vi "SwerveChooseBestAngle.vi"(6 "Current Angle":dbl format="%#_13g", 8 "Target Angle":dbl format="%#_13g", 11 "Power In":dbl) -> (0 "Setpoint Angle":dbl format="%_4g", 2 "Power Out":dbl)   [LabVIEW 2020]
doc: "Based on the Current Angle and the Goal Angle, this VI calulates the signed angular distance. Taking into account the option to invert the direction of the swerve drive motor and always picking the shortest travel distance. The hysteresis prevents undesirable vacillation between angle choices."
panel:
  # "(deg) [-180,+180]"
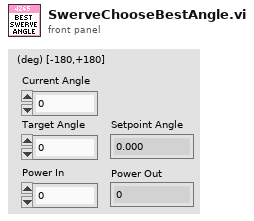
[diagram p1: front panel]
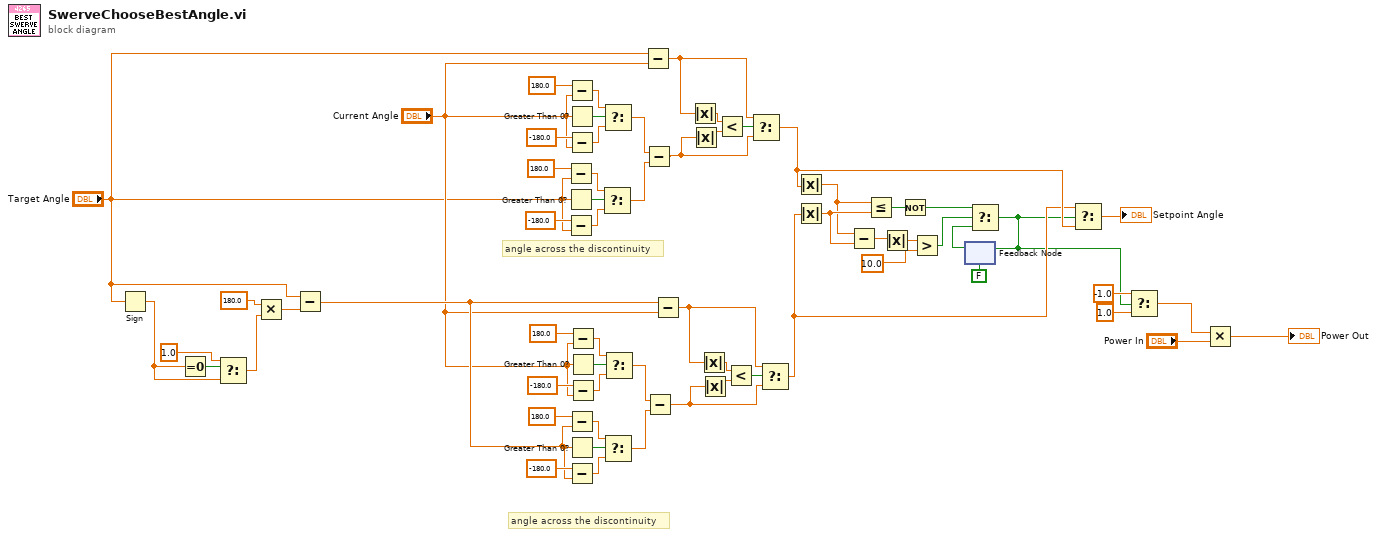
[diagram p0: block diagram]
diagram:
  # "angle across the discontinuity"
  # "angle across the discontinuity"
  n1 = Sign(1:"Target Angle") -> (0:w14:dbl)
  n2 = Equal To 0?(x=w14) -> (x = 0?=w15:bool)
  n3 = Select(t=1.0, s=w15, f=w14) -> (s? t:f=w11:dbl)
  n4 = Multiply(x=180.0 ("y"), y=w11) -> (x*y=w62:dbl)
  n5 = Subtract(x="Target Angle", y=w62) -> (x-y=w36:dbl)
  n6 = Subtract(x=180.0, y="Target Angle") -> (x-y=w24:dbl)
  n7 = Greater Than 0?(x="Target Angle") -> (x > 0?=w26:bool)
  n8 = Subtract(x=-180.0, y="Target Angle") -> (x-y=w22:dbl)
  n9 = Subtract(x=180.0, y="Current Angle") -> (x-y=w29:dbl)
  n10 = Greater Than 0?(x="Current Angle") -> (x > 0?=w31:bool)
  n11 = Subtract(x=-180.0, y="Current Angle") -> (x-y=w27:dbl)
  n12 = Subtract(x=180.0, y=w36) -> (x-y=w45:dbl)
  n13 = Greater Than 0?(x=w36) -> (x > 0?=w47:bool)
  n14 = Subtract(x=-180.0, y=w36) -> (x-y=w43:dbl)
  n15 = Subtract(x=180.0, y="Current Angle") -> (x-y=w51:dbl)
  n16 = Greater Than 0?(x="Current Angle") -> (x > 0?=w53:bool)
  n17 = Subtract(x=-180.0, y="Current Angle") -> (x-y=w49:dbl)
  n18 = Select(t=w24, s=w26, f=w22) -> (s? t:f=w20:dbl)
  n19 = Select(t=w29, s=w31, f=w27) -> (s? t:f=w21:dbl)
  n20 = Select(t=w45, s=w47, f=w43) -> (s? t:f=w41:dbl)
  n21 = Select(t=w51, s=w53, f=w49) -> (s? t:f=w42:dbl)
  n22 = Subtract(x="Target Angle", y="Current Angle") -> (x-y=w32:dbl)
  n23 = Subtract(x=w21, y=w20) -> (x-y=w18:dbl)
  n24 = Subtract(x=w42, y=w41) -> (x-y=w40:dbl)
  n25 = Subtract(x=w36, y="Current Angle") -> (x-y=w37:dbl)
  n26 = Absolute Value(x=w32) -> (abs(x)=w33:dbl)
  n27 = Absolute Value(x=w18) -> (abs(x)=w34:dbl)
  n28 = Absolute Value(x=w37) -> (abs(x)=w38:dbl)
  n29 = Absolute Value(x=w40) -> (abs(x)=w39:dbl)
  n30 = Less?(x=w33, y=w34) -> (x < y?=w35:bool)
  n31 = Less?(x=w38, y=w39) -> (x < y?=w48:bool)
  n32 = Select(t=w32, s=w35, f=w18) -> (s? t:f=w10:dbl)
  n33 = Select(t=w37, s=w48, f=w40) -> (s? t:f=w9:dbl)
  n34 = Absolute Value(x=w10) -> (abs(x)=w54:dbl)
  n35 = Absolute Value(x=w9) -> (abs(x)=w55:dbl)
  n36 = Subtract(x=w54, y=w55) -> (x-y=w58:dbl)
  n37 = Less Or Equal?(x=w54, y=w55) -> (x <= y?=w17:bool)
  n38 = Absolute Value(x=w58) -> (abs(x)=w57:dbl)
  n39 = Not(x=w17) -> (.not. x?=w16:bool)
  n40 = Greater?(x=w57, y=10.0) -> (0:w56:bool)
  n41 = feedback #1(FALSE) -> (w60:bool)
  n42 = Select(t=w16, s=w56, f=w60) -> (s? t:f=w1:bool)
  n43 = feedback-in #1(w1) -> ()
  n44 = Select(t=w9, s=w1, f=w10) -> (s? t:f=→"Setpoint Angle":dbl)
  n45 = Select(t=-1.0, s=w1, f=1.0) -> (s? t:f=w6:dbl)
  n46 = Multiply(x=w6, y="Power In") -> (x*y=→"Power Out":dbl)
